vi "User Guide.vi"() -> ()   [LabVIEW 2021, in "RocketPlot.lvlib"]
uses:
  RocketPlot.lvlib
panel:
  in  "Help":bool
  # "Autosize\nall axes"
  # "Zoom in\ntime axis"
  # "Page\nUp"
  # "Zoom in\ny axis"
  # "Home"
  # "Insert"
  # "Right Click"
  # "Delta values"
  # "Middle Click"
  # "Right Click +Ctrl"
  # "Slive average"
  # "Pan"
  # "Left Click"
  # "Right Click +Shift"
  # "Plot names"
  # "Zoom out\ntime axis"
  # "Page\nDown"
  # "Zoom out\ny axis"
  # "Delete"
  # "Zoom to\nselection"
  # "Tool Tips"
  # "Wheel scroll"
  # "Zoom in/out"
  # "Pan\nin increments"
  # "Zoom actions apply\nto all axes"
  # "Shift"
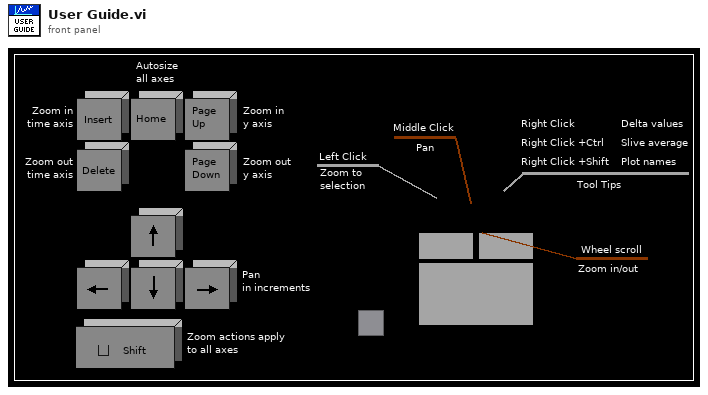
[diagram p1: front panel]
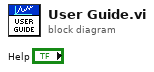
[diagram p0: block diagram]
diagram:
